vi "Start Service.vi"(11 "error in (no error)":errorcluster) -> (15 "error out":errorcluster)   [LabVIEW 2021, in "Migrator.lvlib"]
uses:
  Migrator.lvlib
  Path Functions/Path Functions.lvlib
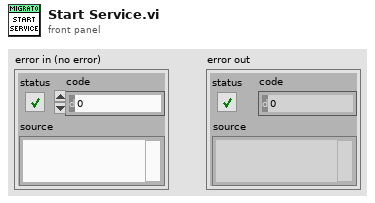
[diagram p1: front panel]
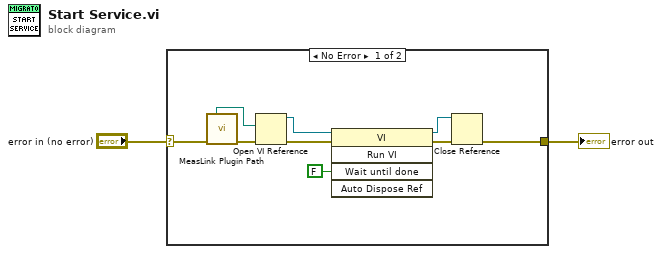
[diagram p0: block diagram]
diagram:
  n1 = case shown="No Error" "error in (no error)" {
    selector: "error in (no error)" -> [w11 w12]
    tunnel: [w3 w12] -> w1
    frame No Error {
      n2 = call "MeasLink Plugin Path.vi"("error in (no error)"=w11) -> ("Run Service"=w10:path, "error out"=w9:errorcluster)  [unwired: 2 in, 11 out]
      n3 = Open VI Reference(vi path=w10, error in (no error)=w9) -> (vi reference=w8:refnum<vi>, error out=w7:errorcluster)  [unwired: 4 in]
      n4 = invoke class="VI" method="Run VI"(reference=w8, error in=w7, "Wait until done"=FALSE ("Wait Until Done")) -> (reference out=w4:refnum<vi>, error out=w5:errorcluster)  [unwired: 2 in, 3 out]
      n5 = Close Reference(reference=w4, error in (no error)=w5) -> (error out=w3:errorcluster)
    }
    frame Error {
    }
  }
  "error out" <- w1
